vi "Check Time.vi"(8 "error in (no error)":errorcluster, 11 "BiStableShutter in":refnum<class "BiStableShutter.lvclass">) -> (0 "error out":errorcluster, 3 "BiStableShutter out":refnum<class "BiStableShutter.lvclass">)   [LabVIEW 2016, in "BiStableShutter.lvclass"]
uses:
  BiStableShutter.lvclass
  Controls/Shutter States.ctl
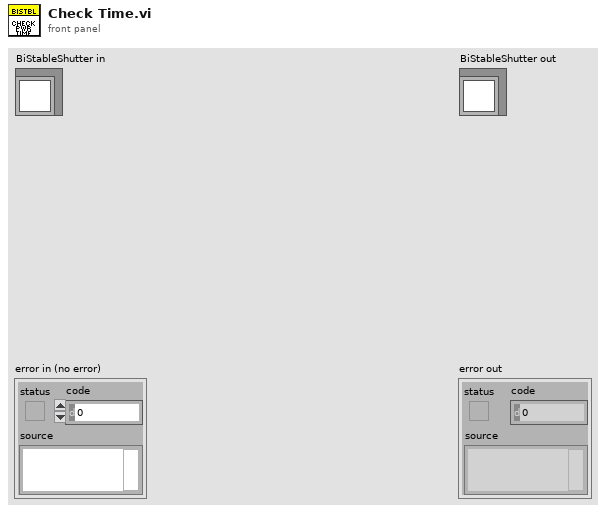
[diagram p1: front panel]
types:
  T1 = typedef "Shutter States.ctl" = enum16{"Open", "Close", "Wait", "Off", "Arm", "Idle"}
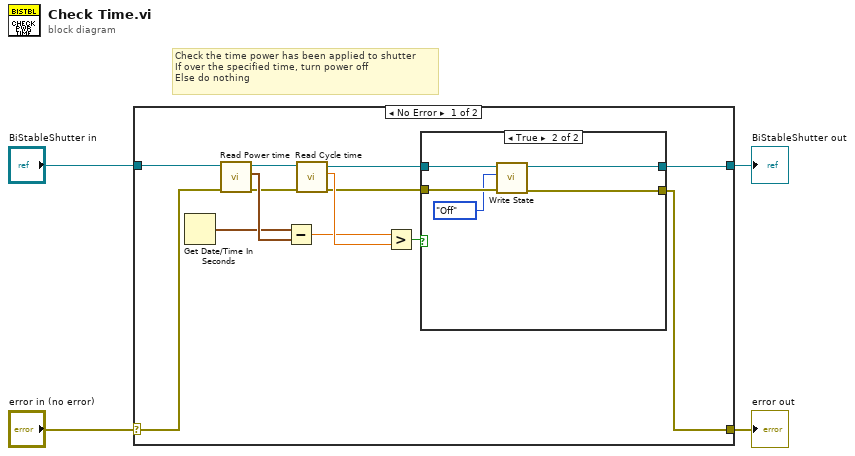
[diagram p0: block diagram]
diagram:
  # "Check the time power has been applied to shutter\nIf over the specified time, turn power off\nElse do nothing"
  n1 = case shown="No Error" "error in (no error)" {
    selector: "error in (no error)" -> [w7 w26]
    tunnel: [w6 w26] -> w3
    tunnel: [w11 w25] -> w1
    tunnel: "BiStableShutter in" -> [w17 w25]
    frame No Error {
      n2 = Get Date/Time In Seconds() -> (seconds since 1Jan1904=w14:timestamp)
      n3 = call-dynamic "Read Power time.vi"("error in (no error)"=w7, "BiStableShutter in"=w17) -> ("error out"=w5:errorcluster, "Power time"=w15:timestamp, "BiStableShutter out"=w16:refnum<class "BiStableShutter.lvclass">)  [unwired: 7 in]
      n4 = Subtract(x=w14, y=w15) -> (x-y=w12:dbl)
      n5 = call-dynamic "Read Cycle time.vi"("error in (no error)"=w5, "BiStableShutter in"=w16) -> ("error out"=w9:errorcluster, "Cycle time"=w13:dbl, "BiStableShutter out"=w10:refnum<class "BiStableShutter.lvclass">)  [unwired: 7 in]
      n6 = Greater?(x=w12, y=w13) -> (0:w8:bool)
      n7 = case shown="True" w8 {
        tunnel: [w19 w24] -> w11
        tunnel: w10 -> [w19 w23]
        tunnel: w9 -> [w18 w22]
        tunnel: [w18 w20] -> w6
        frame False {
        }
        frame True {
          n8 = call-dynamic "Write State.vi"("error in (no error)"=w22, "Set"=Shutter_States."Off", "BiStableShutter in"=w23) -> ("error out"=w20:errorcluster, "BiStableShutter out"=w24:refnum<class "BiStableShutter.lvclass">)  [unwired: 7 in]
        }
      }
    }
    frame Error {
    }
  }
  "error out" <- w3
  "BiStableShutter out" <- w1
